vi "Change FP Window bounds_LV2010.vi"() -> ()   [LabVIEW 2010]
uses:
  <vilib>/Utility/miscctls.llb/LVRectTypeDef.ctl
panel:
  in  "Desired Front Panel Coordinates":T1={"Left"=100, "Top"=200, "Right"=800, "Bottom"=600}
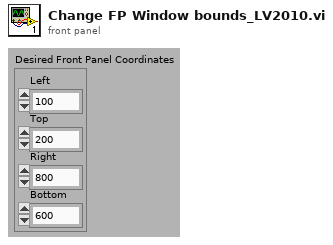
[diagram p1: front panel]
types:
  T1 = typedef "LVRectTypeDef.ctl" = cluster{"Left":i16, "Top":i16, "Right":i16, "Bottom":i16}
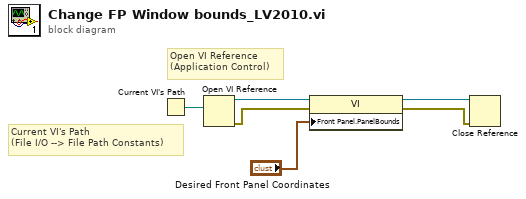
[diagram p0: block diagram]
diagram:
  # "Open VI Reference\n(Application Control)"
  # "Current VI's Path\n(File I/O --> File Path Constants)"
  n1 = Current VI's Path() -> (path=w6:path)
  n2 = Open VI Reference(vi path=w6) -> (vi reference=w5:refnum<vi>, error out=w4:errorcluster)  [unwired: 5 in]
  n3 = property class="VI"(reference=w5, error in=w4, "Front Panel.PanelBounds"="Desired Front Panel Coordinates") -> (reference out=w2:refnum<vi>, error out=w1:errorcluster)
  n4 = Close Reference(reference=w2, error in (no error)=w1) -> ()  [unwired: 1 out]
